vi "7_VI_Latitude_convert.vi"(10 "Latitude (ddmm.mmmmm)":string) -> (1 "Latitude":dbl)   [LabVIEW 2019]
doc: "SubVI der omdanner NMEA string til Latitude værdi\n\nBygget på VI diagram fra dokumentet: \nZED-F9P RTK GPS E2019\nMechatronic challenge group 10\nAarhus University\nThe 21st May 2019"
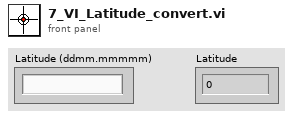
[diagram p1: front panel]
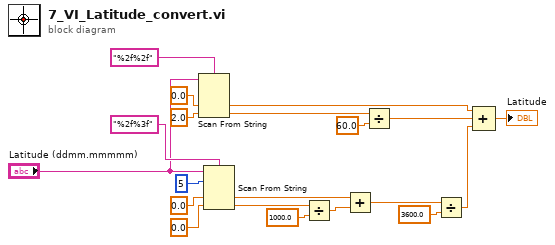
[diagram p0: block diagram]
diagram:
  n1 = Scan From String(format string="%2f%2f", input string="Latitude (ddmm.mmmmm)", default 1=0.0 ("default value 1"), default 2=2.0 ("default value 2")) -> (output 1=w11:dbl, output 2=w12:dbl)  [unwired: 2 in, 3 out]
  n2 = Scan From String(format string="%2f%3f", input string="Latitude (ddmm.mmmmm)", initial scan location=u32 5, default 1=0.0 ("default value 1"), default 2=0.0 ("default value 2")) -> (output 1=w14:dbl, output 2=w15:dbl)  [unwired: 1 in, 3 out]
  n3 = Divide(x=w15, y=1000.0) -> (x/y=w7:dbl)
  n4 = Add(x=w14, y=w7) -> (x+y=w8:dbl)
  n5 = Divide(x=w12, y=60.0) -> (x/y=w9:dbl)
  n6 = Divide(x=w8, y=3600.0) -> (x/y=w10:dbl)
  n7 = Compound Arithmetic op=ADD(w11, w9, w10) -> (→"Latitude":dbl)
